vi "AlignSelection.vi"(7 "Executed on Frontpanel?":bool, 8 "error in (no error)":errorcluster, 9 "Align Type":T1(ring), 10 "Panel Ref in":refnum<vi>, 11 "TopLevelDiagram in":refnum<vi>) -> (0 "error out":errorcluster, 2 "Panel Ref out":refnum<vi>, 3 "TopLevelDiagram out":refnum<vi>)   [LabVIEW 2020, in "Align Elements.lvlib"]
doc: "Align a selectection of elements either on a frontpanel or on a blockdiagram."
uses:
  Align Elements.lvlib
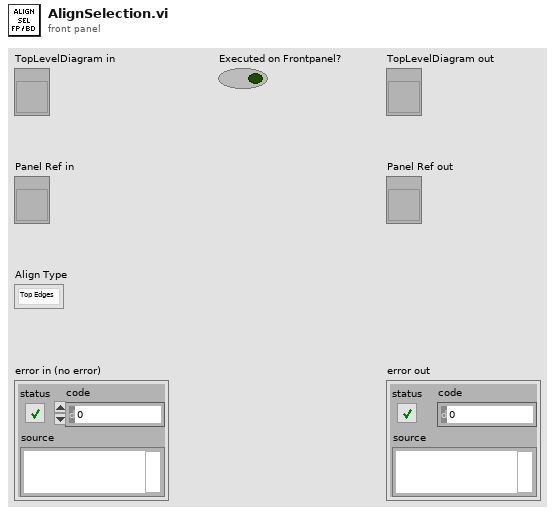
[diagram p1: front panel]
types:
  T1 = enum32{"Top Edges", "Vertical Centers", "Bottom Edges", "Left Edges", "Horizontal Centers", "Right Edges"}
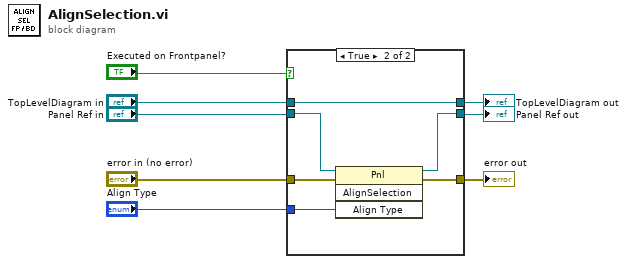
[diagram p0: block diagram]
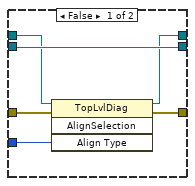
[diagram p2: hidden frame]
diagram:
  n1 = case shown="True" "Executed on Frontpanel?" {
    tunnel: "Align Type" -> [w14 w20]
    tunnel: "TopLevelDiagram in" -> [w12 w19]
    tunnel: [w11 w19] -> w3
    tunnel: "Panel Ref in" -> [w13 w18]
    tunnel: [w13 w17] -> w5
    tunnel: "error in (no error)" -> [w10 w16]
    tunnel: [w9 w15] -> w7
    frame False {
      n2 = invoke class="TopLvlDiag" method="AlignSelection"(reference=w12, error in=w10, "Align Type"=w14) -> (reference out=w11:refnum<vi>, error out=w9:errorcluster)  [unwired: 1 in, 2 out]
    }
    frame True {
      n3 = invoke class="Pnl" method="AlignSelection"(reference=w18, error in=w16, "Align Type"=w20) -> (reference out=w17:refnum<vi>, error out=w15:errorcluster)  [unwired: 1 in, 2 out]
    }
  }
  "error out" <- w7
  "Panel Ref out" <- w5
  "TopLevelDiagram out" <- w3
